vi "Controller Apply Configuration from GUI.vi"(7 "Sync Objects":T12, 8 "error in (no error)":errorcluster, 10 "Configuration Data (GUI to Controller)":T11, 11 "FOFB Configuration":T1={"FOFB Parameters"={"Network"={"FOFB Controller IP"="", "LNLS Control Network IP"="", "LNLS Control Network Power Supplies TCP Port"=0, "LNLS Control Network FOFB Configuration TCP Port"=0, "LNLS Control Network BPMs TCP Port"=0, "Data Server TCP Port"=0, "Monitoring Data TCP Port"=0, "Configuration GUI TCP Port"=0, "Storage Data TCP Port"=0, "Fast Command TCP Port"=0, "TCP Listening Timeout"=0, "Request Setpoints Rate"=0}, "Fast Acquisition"={"Acquisition Period"=0, "Data Buffer Size"=0, "Monitoring Period"=0}, "Response Matrix Measurement"={"Step Amplitude"=0.0, "Time Between Steps"=0, "Step Duration"=0, "Number of Averages"=0}, "Correction Algorithm"={"Correction Period"=0, "Reference Orbit Path"=path "", "Response Matrix Path"=path "", "Correction Matrix Path"=path "", "PID Horizontal Gain"=0.0, "PID Vertical Gain"=0.0, "PID Horizontal Integral Time"=0.0, "PID Vertical Integral Time"=0.0, "PID Horizontal Derivative Time"=0.0, "PID Vertical Derivative Time"=0.0, "Beam Current FOFB Threshold"=0.0, "Decouple H-V"=FALSE, "Use Additional BPM LPF"=FALSE, "BPM LPF Cutoff"=0.0}, "Acquisition Network"=[], "Actuation Network"=[]}, "Number of Acquisition Chassis"=0, "Number of Actuation Chassis"=0, "Number of BPM Readings"=0, "BPM Reading Names"=[], "Selected BPM Readings"=[0, 1, 2, 3, 4, 5, 6, 7, 8, 9, 10, 11, 12, 13, 14, 15, 16, 17, 18, 19, 20, 21, 22, 23, 24, 25, 26, 27, 28, 29, 30, 31, 32, 33, 34, 35, 36, 37, 38, 39, 40, 41, 42, 43, 44, 45, 46, 47, 48, 49], "Number of Correctors"=0, "Corrector Names"=[], "Selected Correctors"=[0, 1, 2, 3, 4, 5, 6, 7, 8, 9, 10, 11, 12, 13, 14, 15, 16, 17, 18, 19, 20, 21, 22, 23, 24, 25, 26, 27, 28, 29, 30, 31, 32, 33, 34, 35, 36, 37, 38, 39, 40, 41, 42, 43, 44, 45, 46, 47, 48, 49], "Reference Orbit"=[], "Response Matrix"=[], "Correction Matrix"=[], "Acquisition Chassis Names"=[], "Actuation Chassis Names"=[], "Acquisition Variables"=[], "Actuation Variables"=[], "PS Matrix Mapping"=[], "Inverse PS Matrix Mapping"=[], "BPM Matrix Mapping"=[], "Inverse BPM Matrix Mapping"=[], "Response Matrix Beam Energy (MeV)"=0.0, "PID Parameters"=[], "BPM Planes"=[], "Corrector Planes"=[], "RMM Step Factor"=[]}) -> (0 "error out":errorcluster, 2 "Configuration Change Acknowledge (Controller to GUI)":T10)   [LabVIEW 2011, in "Controller VIs.lvlib"]
uses:
  Controller VIs.lvlib
  Types Definitions/Type Synchronization Objects.ctl
  Types Definitions/Type Blocking Synchronization Objects.ctl
  Types Definitions/Type Monitoring Data.ctl
  Types Definitions/Type Operation Mode State.ctl
  Types Definitions/Type Diagnostics Data.ctl
  Types Definitions/Type CPU Loads Array.ctl
  Types Definitions/Type CPU Loads.ctl
  Types Definitions/Type Non-blocking Synchronization Objects.ctl
  Types Definitions/Type FOFB Variables.ctl
  Types Definitions/Type Actuation State.ctl
  Types Definitions/Type Configuration Data (GUI to Controller).ctl
  Types Definitions/Type FOFB Parameters.ctl
  Types Definitions/Type Network Configuration.ctl
  Types Definitions/Type FA Configuration.ctl
  Types Definitions/Type Response Matrix Measurement Configuration.ctl
  Types Definitions/Type Correction Algorithm Configuration.ctl
  Types Definitions/Type Acquisition Network Configuration.ctl
  Types Definitions/Type Actuation Network Configuration.ctl
  Types Definitions/Type Configuration Change Acknowledge (Controller to GUI).ctl
  Types Definitions/Type FOFB Configuration.ctl
  Types Definitions/Type PID Parameters.ctl
  Type Definitions.lvlib
  XML VIs.lvlib
  File VIs.lvlib
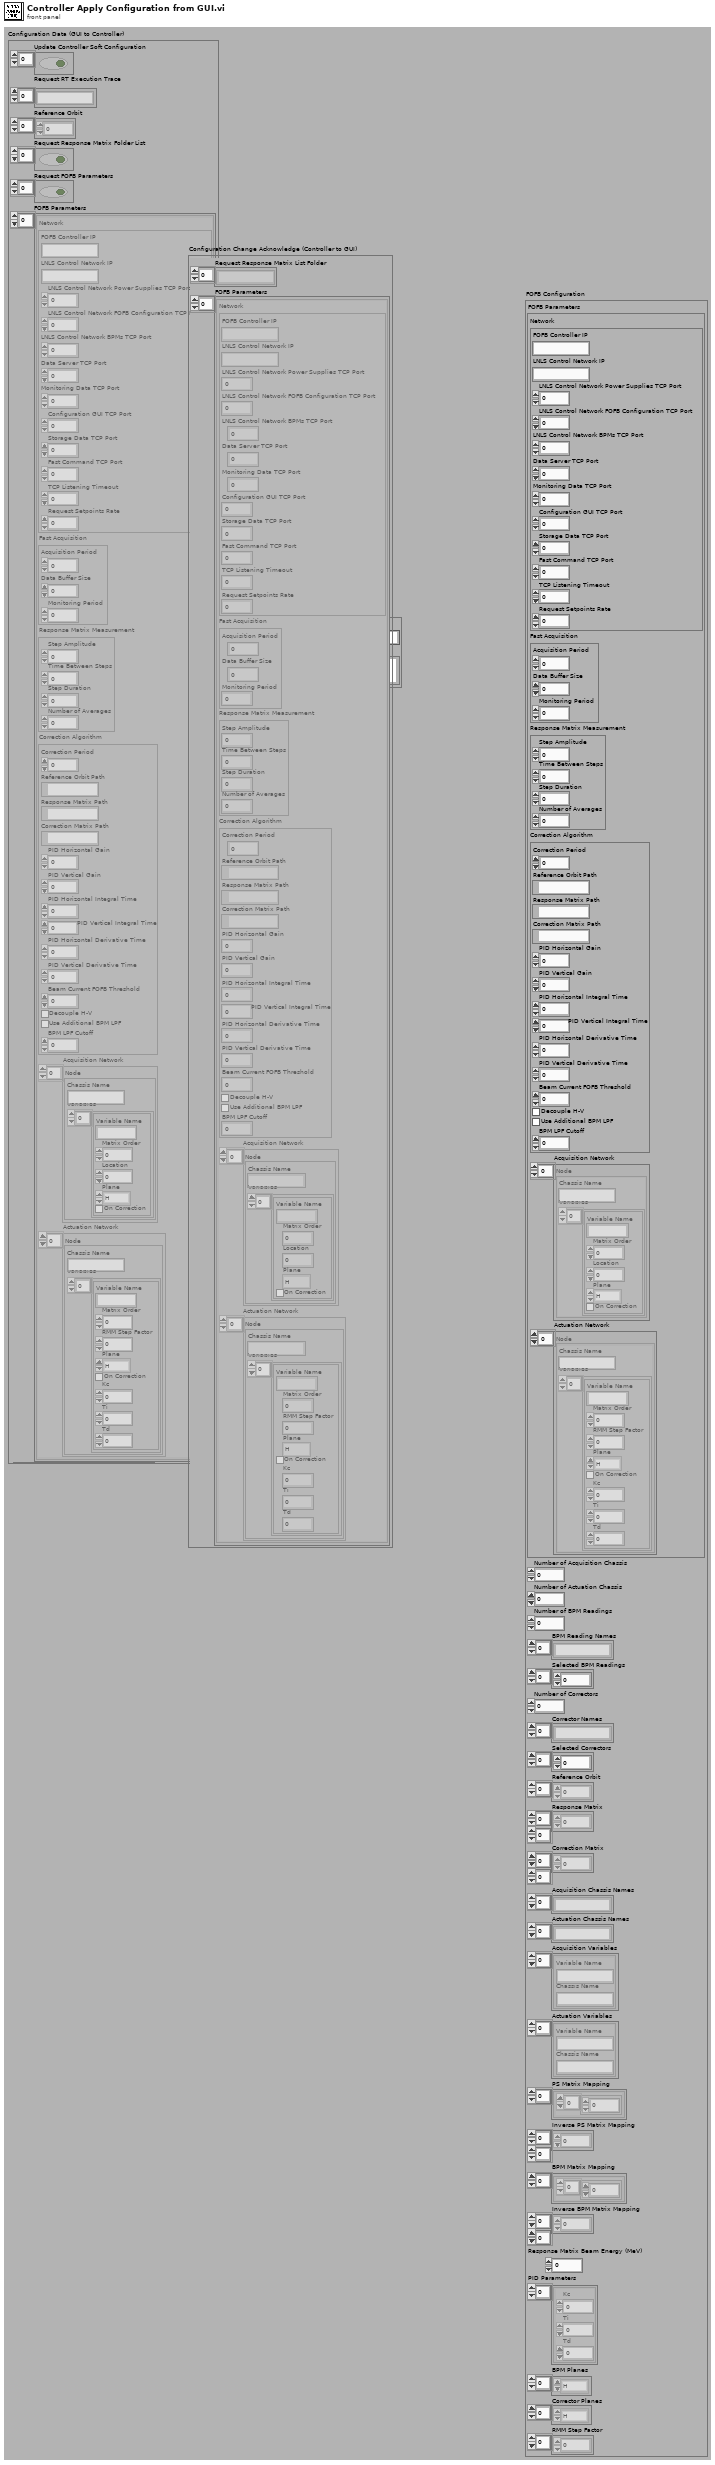
[diagram p1: front panel]
types:
  T1 = typedef "Type Definitions.lvlib/Type FOFB Configuration.ctl" = cluster{"FOFB Parameters":T2, "Number of Acquisition Chassis":i32, "Number of Actuation Chassis":i32, "Number of BPM Readings":i32, "BPM Reading Names":string[], "Selected BPM Readings":u32[], "Number of Correctors":i32, "Corrector Names":string[], "Selected Correctors":u32[], "Reference Orbit":dbl[], "Response Matrix":dbl[][], "Correction Matrix":dbl[][], "Acquisition Chassis Names":string[], "Actuation Chassis Names":string[], "Acquisition Variables":cluster{"Variable Name":string, "Chassis Name":string}[], "Actuation Variables":cluster{"Variable Name":string, "Chassis Name":string}[], "PS Matrix Mapping":cluster{u32[]}[], "Inverse PS Matrix Mapping":u32[][], "BPM Matrix Mapping":cluster{u32[]}[], "Inverse BPM Matrix Mapping":u32[][], "Response Matrix Beam Energy (MeV)":dbl, "PID Parameters":T9[], "BPM Planes":enum8{"H", "V"}[], "Corrector Planes":enum8{"H", "V"}[], "RMM Step Factor":dbl[]}
  T2 = typedef "Type Definitions.lvlib/Type FOFB Parameters.ctl" = cluster{"Network":T3, "Fast Acquisition":T4, "Response Matrix Measurement":T5, "Correction Algorithm":T6, "Acquisition Network":T7, "Actuation Network":T8}
  T3 = typedef "Type Definitions.lvlib/Type Network Configuration.ctl" = cluster{"FOFB Controller IP":string, "LNLS Control Network IP":string, "LNLS Control Network Power Supplies TCP Port":u16, "LNLS Control Network FOFB Configuration TCP Port":u16, "LNLS Control Network BPMs TCP Port":u16, "Data Server TCP Port":u16, "Monitoring Data TCP Port":u16, "Configuration GUI TCP Port":u16, "Storage Data TCP Port":u16, "Fast Command TCP Port":u16, "TCP Listening Timeout":i32, "Request Setpoints Rate":u16}
  T4 = typedef "Type Definitions.lvlib/Type FA Configuration.ctl" = cluster{"Acquisition Period":u32, "Data Buffer Size":u32, "Monitoring Period":u32}
  T5 = typedef "Type Definitions.lvlib/Type Response Matrix Measurement Configuration.ctl" = cluster{"Step Amplitude":dbl, "Time Between Steps":u32, "Step Duration":u32, "Number of Averages":u32}
  T6 = typedef "Type Definitions.lvlib/Type Correction Algorithm Configuration.ctl" = cluster{"Correction Period":u32, "Reference Orbit Path":path, "Response Matrix Path":path, "Correction Matrix Path":path, "PID Horizontal Gain":dbl, "PID Vertical Gain":dbl, "PID Horizontal Integral Time":dbl, "PID Vertical Integral Time":dbl, "PID Horizontal Derivative Time":dbl, "PID Vertical Derivative Time":dbl, "Beam Current FOFB Threshold":dbl, "Decouple H-V":bool, "Use Additional BPM LPF":bool, "BPM LPF Cutoff":dbl}
  T7 = typedef "Type Definitions.lvlib/Type Acquisition Network Configuration.ctl" = cluster{"Chassis Name":string, "Variables":cluster{"Variable Name":string, "Matrix Order":u32, "Location":dbl, "Plane":enum8{"H", "V"}, "On Correction":bool}[]}[]
  T8 = typedef "Type Definitions.lvlib/Type Actuation Network Configuration.ctl" = cluster{"Chassis Name":string, "Variables":cluster{"Variable Name":string, "Matrix Order":u32, "RMM Step Factor":dbl, "Plane":enum8{"H", "V"}, "On Correction":bool, "Kc":dbl, "Ti":dbl, "Td":dbl}[]}[]
  T9 = typedef "Type Definitions.lvlib/Type PID Parameters.ctl" = cluster{"Kc":fxp<+/-,16,8>, "Ti":fxp<+/-,16,8>, "Td":fxp<+/-,16,8>}
  T10 = typedef "Type Definitions.lvlib/Type Configuration Change Acknowledge (Controller to GUI).ctl" = cluster{"Request Response Matrix List Folder":string[], "FOFB Parameters":T2[]}
  T11 = typedef "Type Definitions.lvlib/Type Configuration Data (GUI to Controller).ctl" = cluster{"Update Controller Soft Configuration":bool[], "Request RT Execution Trace":string[], "Reference Orbit":dbl[], "Request Response Matrix Folder List":bool[], "Request FOFB Parameters":bool[], "FOFB Parameters":T2[]}
  T12 = typedef "Type Definitions.lvlib/Type Synchronization Objects.ctl" = cluster{"Blocking":T13, "Non-blocking":T14}
  T13 = typedef "Type Definitions.lvlib/Type Blocking Synchronization Objects.ctl" = cluster{"RMM Start FIFO":refnum<k33>, "Monitoring Data Notifier":refnum<notifier>, "Storage Data FIFO":refnum<queue>, "Operation Mode Change Request FIFO":refnum<k33>, "Monitoring BPM and PS Data FIFO":refnum<k33>, "FA BPM and PS Data FIFO":refnum<k33>, "PS Manual Setpoints FIFO":refnum<k33>, "PS RMM Setpoints FIFO":refnum<k33>, "FOFB Controller Errors FIFO ":refnum<k33>, "FOFB Status In Notifier":refnum<notifier>, "FOFB Status Out Notifier":refnum<notifier>, "PS Configuration Status In Notifier":refnum<notifier>, "PS Configuration Status Out Notifier":refnum<notifier>, "BPM Configuration Status In Notifier":refnum<notifier>, "BPM Configuration Status Out Notifier":refnum<notifier>, "RT Trace Request Queue":refnum<queue>, "BPM and PS Modified Values":refnum<k33>}
  T14 = typedef "Type Definitions.lvlib/Type Non-blocking Synchronization Objects.ctl" = cluster{"Stop Controller Notifier":refnum<notifier>, "Stop Controller (Time-Critical Loop) FIFO":refnum<k33>, "RMM Finished FIFO":refnum<k33>, "RMM Stop FIFO":refnum<k33>, "FOFB Variables Queue":refnum<queue>, "Diagnostics Data Notifier":refnum<notifier>, "Diagnostics Data (Time-Critical Loop) FIFO":refnum<k33>, "Actuation State Change Request FIFO":refnum<k33>}
  T15 = typedef "Type Definitions.lvlib/Type FOFB Variables.ctl" = cluster{"Correction Period":u32, "Reference Orbit":dbl[], "Response Matrix":dbl[][], "Correction Matrix":dbl[][], "Decouple H-V":bool, "PID Horizontal Gain":dbl, "PID Vertical Gain":dbl, "PID Horizontal Integral Time":dbl, "PID Vertical Integral Time":dbl, "PID Horizontal Derivative Time":dbl, "PID Vertical Derivative Time":dbl, "Selected BPM Readings":u32[], "Selected Correctors":u32[], "BPM Planes":enum8{"H", "V"}[], "Corrector Planes":enum8{"H", "V"}[], "Beam Current FOFB Threshold":dbl, "Response Matrix Beam Energy (MeV)":dbl, "Fast Command Enabled":bool}
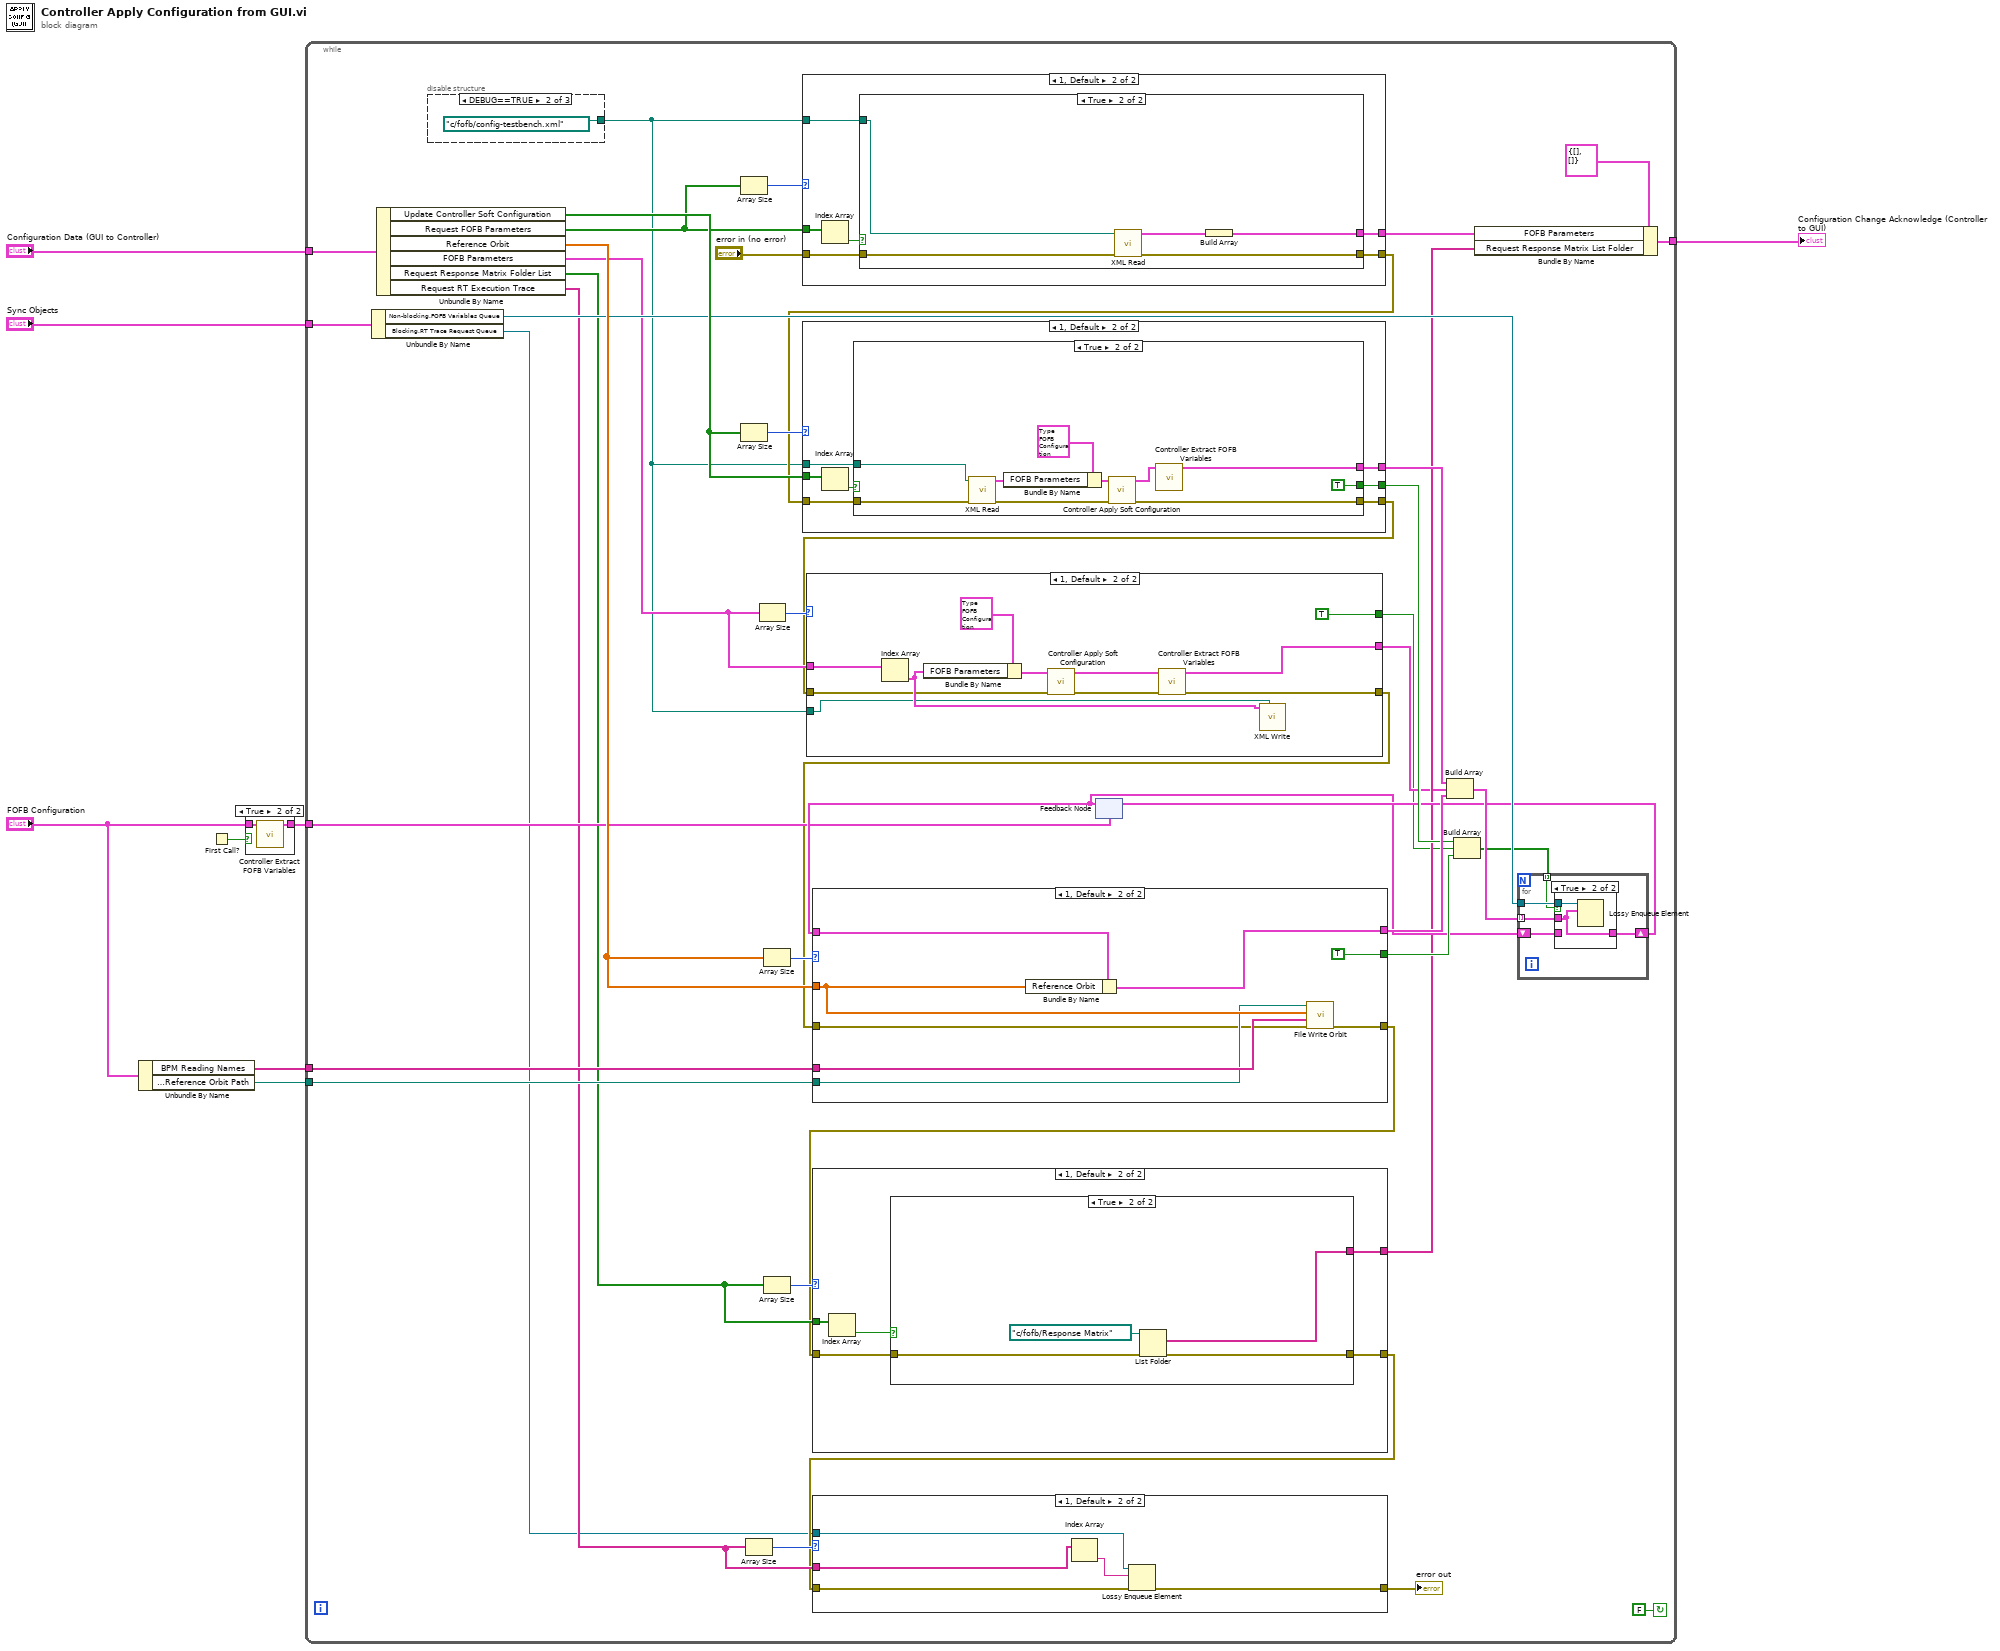
[diagram p0: block diagram]
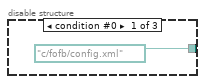
[diagram p4: hidden frame]
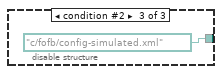
[diagram p5: hidden frame]
diagram:
  n1 = Unbundle By Name("FOFB Configuration") -> ("BPM Reading Names"=w2:string[], "FOFB Parameters.Correction Algorithm.Reference Orbit Path"=w1:path)
  n2 = First Call?() -> (First Call?: T/F=w5:bool)
  n3 = case shown="True" w5 {
    tunnel: "FOFB Configuration" -> [_ w10]
    tunnel: [_ w9] -> w4
    frame False {
    }
    frame True {
      n4 = call "Controller Extract FOFB Variables.vi"("FOFB Configuration"=w10) -> ("FOFB Variables"=w9:T15)  [unwired: 9 in, 1 out]
    }
  }
  n5 = while {
    tunnel: "Sync Objects" -> [w52]
    tunnel: "Configuration Data (GUI to Controller)" -> [w51]
    tunnel: [w42] -> w6
    tunnel: w4 -> [w30]
    tunnel: w2 -> [w29]
    tunnel: w1 -> [w28]
    stop <- FALSE continue-if-true
    n6 = Unbundle By Name(w52) -> ("Non-blocking.FOFB Variables Queue"=w41:refnum<queue>, "Blocking.RT Trace Request Queue"=w18:refnum<queue>)
    n7 = Unbundle By Name(w51) -> ("Update Controller Soft Configuration"=w48:bool[], "Request FOFB Parameters"=w46:bool[], "Reference Orbit"=w43:dbl[], "FOFB Parameters"=w16:T2[], "Request Response Matrix Folder List"=w26:bool[], "Request RT Execution Trace"=w21:string[])
    n8 = disable-structure shown="DEBUG==TRUE" {
      disable-tunnel: [path "c:/fofb/config.xml" ("Configuration File Path") path "c:/fofb/config-testbench.xml" ("Configuration File Path") path "c:/fofb/config-simulated.xml" ("Configuration File Path")] -> w14
      frame condition #0 {
      }
      frame condition #1 (active) {
      }
      frame condition #2 {
      }
    }
    n9 = Array Size(array=w46) -> (size(s)=w47:i32)
    n10 = Array Size(array=w48) -> (size(s)=w49:i32)
    n11 = Array Size(array=w21) -> (size(s)=w22:i32)
    n12 = Array Size(array=w16) -> (size(s)=w17:i32)
    n13 = Array Size(array=w43) -> (size(s)=w44:i32)
    n14 = Array Size(array=w26) -> (size(s)=w27:i32)
    n15 = case shown="1, Default" w47 {
      tunnel: w46 -> [_ w109]
      tunnel: "error in (no error)" -> [w103 w107]
      tunnel: [w103 w106] -> w40
      tunnel: [_ w105] -> w45
      tunnel: w14 -> [_ w104]
      frame 0 {
      }
      frame 1, Default {
        n16 = Index Array(array=w109) -> (element=w108:bool)  [unwired: 1 in]
        n17 = case shown="True" w108 {
          tunnel: w107 -> [w110 w115]
          tunnel: [w110 w114] -> w106
          tunnel: [_ w113] -> w105
          tunnel: w104 -> [_ w111]
          frame False {
          }
          frame True {
            n18 = call "XML Read.vi"("error in"=w115, "XML File Path In"=w111) -> ("error out"=w114:errorcluster, "FOFB Parameters"=w112:T2)  [unwired: 8 in]
            n19 = Build Array(w112) -> (w113:T2[])
          }
        }
      }
    }
    n20 = case shown="1, Default" w49 {
      tunnel: w48 -> [_ w123]
      tunnel: w40 -> [w116 w121]
      tunnel: [w116 w119] -> w12
      tunnel: [_ w120] -> w39
      tunnel: [_ w118] -> w37
      tunnel: w14 -> [_ w117]
      frame 0 {
      }
      frame 1, Default {
        n21 = Index Array(array=w123) -> (element=w122:bool)  [unwired: 1 in]
        n22 = case shown="True" w122 {
          tunnel: w121 -> [w124 w131]
          tunnel: [w124 w128] -> w119
          tunnel: [_ w127] -> w120
          tunnel: [_ TRUE] -> w118
          tunnel: w117 -> [_ w125]
          frame False {
          }
          frame True {
            n23 = call "XML Read.vi"("error in"=w131, "XML File Path In"=w125) -> ("error out"=w134:errorcluster, "FOFB Parameters"=w132:T2)  [unwired: 8 in]
            n24 = Bundle By Name(cluster=T1 {"FOFB Parameters"={"Network"={"FOFB Controller IP"="", "LNLS Control Network IP"="", "LNLS Control Network Power Supplies TCP Port"=0, "LNLS Control Network FOFB Configuration TCP Port"=0, "LNLS Control Network BPMs TCP Port"=0, "Data Server TCP Port"=0, "Monitoring Data TCP Port"=0, "Configuration GUI TCP Port"=0, "Storage Data TCP Port"=0, "Fast Command TCP Port"=0, "TCP Listening Timeout"=0, "Request Setpoints Rate"=0}, "Fast Acquisition"={"Acquisition Period"=0, "Data Buffer Size"=0, "Monitoring Period"=0}, "Response Matrix Measurement"={"Step Amplitude"=0.0, "Time Between Steps"=0, "Step Duration"=0, "Number of Averages"=0}, "Correction Algorithm"={"Correction Period"=0, "Reference Orbit Path"=path "", "Response Matrix Path"=path "", "Correction Matrix Path"=path "", "PID Horizontal Gain"=0.0, "PID Vertical Gain"=0.0, "PID Horizontal Integral Time"=0.0, "PID Vertical Integral Time"=0.0, "PID Horizontal Derivative Time"=0.0, "PID Vertical Derivative Time"=0.0, "Beam Current FOFB Threshold"=0.0, "Decouple H-V"=FALSE, "Use Additional BPM LPF"=FALSE, "BPM LPF Cutoff"=0.0}, "Acquisition Network"=[], "Actuation Network"=[]}, "Number of Acquisition Chassis"=0, "Number of Actuation Chassis"=0, "Number of BPM Readings"=0, "BPM Reading Names"=[], "Selected BPM Readings"=[], "Number of Correctors"=0, "Corrector Names"=[], "Selected Correctors"=[], "Reference Orbit"=[], "Response Matrix"=[], "Correction Matrix"=[], "Acquisition Chassis Names"=[], "Actuation Chassis Names"=[], "Acquisition Variables"=[], "Actuation Variables"=[], "PS Matrix Mapping"=[], "Inverse PS Matrix Mapping"=[], "BPM Matrix Mapping"=[], "Inverse BPM Matrix Mapping"=[], "Response Matrix Beam Energy (MeV)"=0.0, "PID Parameters"=[], "BPM Planes"=[], "Corrector Planes"=[], "RMM Step Factor"=[]}, "FOFB Parameters"=w132) -> (w133:T1)
            n25 = call "Controller Apply Soft Configuration.vi"("error in (no error)"=w134, "FOFB Configuration"=w133) -> ("error out"=w128:errorcluster, "FOFB Configuration"=w130:T1)  [unwired: 8 in]
            n26 = call "Controller Extract FOFB Variables.vi"("FOFB Configuration"=w130) -> ("FOFB Variables"=w127:T15)  [unwired: 9 in, 1 out]
          }
        }
      }
    }
    n27 = case shown="1, Default" w17 {
      tunnel: w16 -> [_ w64]
      tunnel: [_ w60] -> w15
      tunnel: w14 -> [_ w58]
      tunnel: [_ TRUE] -> w13
      tunnel: w12 -> [w53 w56]
      tunnel: [w53 w54] -> w11
      frame 0 {
      }
      frame 1, Default {
        n28 = Index Array(array=w64) -> (element=w59:T2)  [unwired: 1 in]
        n29 = Bundle By Name(cluster=T1 {"FOFB Parameters"={"Network"={"FOFB Controller IP"="", "LNLS Control Network IP"="", "LNLS Control Network Power Supplies TCP Port"=0, "LNLS Control Network FOFB Configuration TCP Port"=0, "LNLS Control Network BPMs TCP Port"=0, "Data Server TCP Port"=0, "Monitoring Data TCP Port"=0, "Configuration GUI TCP Port"=0, "Storage Data TCP Port"=0, "Fast Command TCP Port"=0, "TCP Listening Timeout"=0, "Request Setpoints Rate"=0}, "Fast Acquisition"={"Acquisition Period"=0, "Data Buffer Size"=0, "Monitoring Period"=0}, "Response Matrix Measurement"={"Step Amplitude"=0.0, "Time Between Steps"=0, "Step Duration"=0, "Number of Averages"=0}, "Correction Algorithm"={"Correction Period"=0, "Reference Orbit Path"=path "", "Response Matrix Path"=path "", "Correction Matrix Path"=path "", "PID Horizontal Gain"=0.0, "PID Vertical Gain"=0.0, "PID Horizontal Integral Time"=0.0, "PID Vertical Integral Time"=0.0, "PID Horizontal Derivative Time"=0.0, "PID Vertical Derivative Time"=0.0, "Beam Current FOFB Threshold"=0.0, "Decouple H-V"=FALSE, "Use Additional BPM LPF"=FALSE, "BPM LPF Cutoff"=0.0}, "Acquisition Network"=[], "Actuation Network"=[]}, "Number of Acquisition Chassis"=0, "Number of Actuation Chassis"=0, "Number of BPM Readings"=0, "BPM Reading Names"=[], "Selected BPM Readings"=[], "Number of Correctors"=0, "Corrector Names"=[], "Selected Correctors"=[], "Reference Orbit"=[], "Response Matrix"=[], "Correction Matrix"=[], "Acquisition Chassis Names"=[], "Actuation Chassis Names"=[], "Acquisition Variables"=[], "Actuation Variables"=[], "PS Matrix Mapping"=[], "Inverse PS Matrix Mapping"=[], "BPM Matrix Mapping"=[], "Inverse BPM Matrix Mapping"=[], "Response Matrix Beam Energy (MeV)"=0.0, "PID Parameters"=[], "BPM Planes"=[], "Corrector Planes"=[], "RMM Step Factor"=[]}, "FOFB Parameters"=w59) -> (w62:T1)
        n30 = call "Controller Apply Soft Configuration.vi"("error in (no error)"=w56, "FOFB Configuration"=w62) -> ("error out"=w55:errorcluster, "FOFB Configuration"=w61:T1)  [unwired: 8 in]
        n31 = call "Controller Extract FOFB Variables.vi"("error in (no error)"=w55, "FOFB Configuration"=w61) -> ("error out"=w54:errorcluster, "FOFB Variables"=w60:T15)  [unwired: 8 in]
        n32 = call "XML Write.vi"("XML File Path Write"=w58, "FOFB Parameters"=w59) -> ()  [unwired: 8 in, 2 out]
      }
    }
    n33 = feedback #1(w30) -> (w32:T15)
    n34 = case shown="1, Default" w44 {
      tunnel: w43 -> [_ w99]
      tunnel: w11 -> [w94 w96]
      tunnel: [w94 w95] -> w25
      tunnel: w32 -> [w93 w102]
      tunnel: [_ TRUE] -> w36
      tunnel: [w93 w100] -> w38
      tunnel: w29 -> [_ w98]
      tunnel: w28 -> [_ w97]
      frame 0 {
      }
      frame 1, Default {
        n35 = Bundle By Name(cluster=w102, "Reference Orbit"=w99) -> (w100:T15)
        n36 = call "File Write Orbit.vi"("error in (no error)"=w96, "BPM Reading Names"=w98, "Orbit"=w99, "file path (dialog if empty)"=w97) -> ("error out"=w95:errorcluster)  [unwired: 6 in]
      }
    }
    n37 = case shown="1, Default" w27 {
      tunnel: w25 -> [w74 w77]
      tunnel: [w74 w76] -> w20
      tunnel: w26 -> [_ w79]
      tunnel: [_ w75] -> w23
      frame 0 {
      }
      frame 1, Default {
        n38 = Index Array(array=w79) -> (element=w78:bool)  [unwired: 1 in]
        n39 = case shown="True" w78 {
          tunnel: w77 -> [w80 w83]
          tunnel: [w80 w82] -> w76
          tunnel: [_ w81] -> w75
          frame False {
          }
          frame True {
            n40 = List Folder(path=path "c:/fofb/Response Matrix", error in=w83) -> (filenames=w81:string[], error out=w82:errorcluster)  [unwired: 2 in, 2 out]
          }
        }
      }
    }
    n41 = case shown="1, Default" w22 {
      tunnel: w21 -> [_ w73]
      tunnel: w18 -> [_ w71]
      tunnel: w20 -> [w68 w70]
      tunnel: [w68 w69] -> w19
      frame 0 {
      }
      frame 1, Default {
        n42 = Index Array(array=w73) -> (element=w72:string)  [unwired: 1 in]
        n43 = Lossy Enqueue Element(queue=w71, element=w72, error in (no error)=w70) -> (error out=w69:errorcluster)  [unwired: 3 out]
      }
    }
    "error out" <- w19
    n44 = Build Array(w39, w15, w38) -> (w35:T15[])
    n45 = Build Array(w37, w13, w36) -> (w34:bool[])
    n46 = Bundle By Name(cluster=T10 {"Request Response Matrix List Folder"=[], "FOFB Parameters"=[]} ("Configuration Change Acknowledge (Controller to GUI)"), "FOFB Parameters"=w45, "Request Response Matrix List Folder"=w23) -> (w42:T10)
    n47 = for {
      tunnel: w41 -> [w89]
      tunnel: w35 -> [w87] mode=indexing
      tunnel: w34 -> [w88] mode=indexing
      shift-right: [w86] -> w33
      shift-left: w32 -> [w85]
      n48 = case shown="True" w88 {
        tunnel: w89 -> [_ w92]
        tunnel: w87 -> [_ w91]
        tunnel: [w90 w91] -> w86
        tunnel: w85 -> [w90 _]
        frame False {
        }
        frame True {
          n49 = Lossy Enqueue Element(queue=w92, element=w91) -> ()  [unwired: 1 in, 4 out]
        }
      }
    }
    n50 = feedback-in #1(w33) -> ()
  }
  "Configuration Change Acknowledge (Controller to GUI)" <- w6
